vi "sub_log-path.vi"() -> (2 "result path":path, 3 "log path":path)   [LabVIEW 2019]
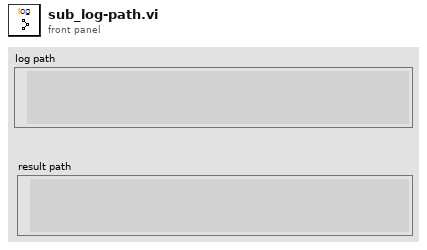
[diagram p1: front panel]
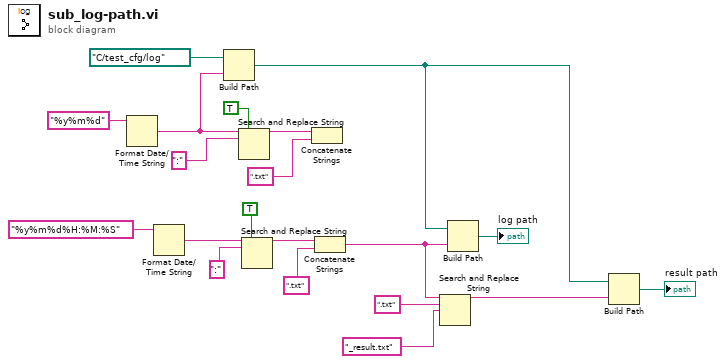
[diagram p0: block diagram]
diagram:
  n1 = Format Date/Time String(time format string (%c)="%y%m%d" ("시간 포맷 문자열 (%c)")) -> (date/time string=w8:string)  [unwired: 2 in]
  n2 = Format Date/Time String(time format string (%c)="%y%m%d%H:%M:%S" ("시간 포맷 문자열 (%c)")) -> (date/time string=w9:string)  [unwired: 2 in]
  n3 = Build Path(base path=path "C:/test_cfg/log", name or relative path=w8) -> (appended path=w3:path)
  n4 = Search and Replace String(replace all?=TRUE ("replace all? (F)"), input string=w8, search string=":") -> (result string=w18:string)  [unwired: 5 in, 3 out]
  n5 = Search and Replace String(replace all?=TRUE ("replace all? (F)"), input string=w9, search string=":") -> (result string=w12:string)  [unwired: 5 in, 3 out]
  n6 = Concatenate Strings(w18, ".txt" ("string")) -> ()  [unwired: 1 out]
  n7 = Concatenate Strings(w12, ".txt" ("string")) -> (w6:string)
  n8 = Search and Replace String(input string=w6, search string=".txt", replace string="_result.txt" ("search string")) -> (result string=w2:string)  [unwired: 5 in, 3 out]
  n9 = Build Path(base path=w3, name or relative path=w6) -> (appended path=→"log path":path)
  n10 = Build Path(base path=w3, name or relative path=w2) -> (appended path=→"result path":path)
